vi "nanocal-frontend-server.vi"() -> ()   [LabVIEW 2020]
uses:
  icicle.ctl
  publisher action.ctl
  NanoCalLib 20210521/NanoCalLib.lvlibp
  NanoCalLib 20210521/MCL.lvlibp/SynkTek FPGA/FPGA_SharedResources/FPGASharedResources_Lockin_Typedef.ctl
  NanoCalLib 20210521/MCL.lvlibp/SynkTek FPGA/FPGA_SharedResources/FPGA_SharedResources.lvlib
  NanoCalLib 20210521/MCL.lvlibp
  NanoCalLib 20210521/MCL.lvlibp/SynkTek FPGA/FPGA_SharedResources/FPGASharedResources_Readings_ReadingChannelTypedef.ctl
  NanoCalLib 20210521/MCL.lvlibp/SynkTek FPGA/FPGA_SharedResources/FPGASharedResources_PhaseType_Typedef.ctl
panel:
  in  "Tab Control":enum32{"Page 1", "Page 2"}(tab)
  in  "wait (ms)":u32=50
  out "nanocal data":T1[](array[typedef])=[{"name"="frequency", "units"="Hz", "data"=22.999983439900642}, {"name"="Cs/T", "units"="J/K^2", "data"=3.7739249893269324e-24}, {"name"="Ts", "units"="K", "data"=0.01038672245174747}, {"name"="Ts^2", "units"="K^2", "data"=0.00010788400328963498}, {"name"="Tr", "units"="K", "data"=0.010160855980464388}, {"name"="Cs", "units"="J/K", "data"=3.9198711417852884e-26}, {"name"="Cr", "units"="J/K", "data"=-2.0417082109734875e-18}, {"name"="Ks", "units"="W/K", "data"=2.527872170547633e-23}, {"name"="Kr", "units"="W/K", "data"=3.911459306754245e-15}, {"name"="Rs-therm", "units"="Ohm", "data"=81348.62911437088}, {"name"="Rr-therm", "units"="Ohm", "data"=196009.13306498667}, {"name"="Cr/T", "units"="J/K^2", "data"=-2.0093860348960226e-16}, {"name"="dlogR/dlogT -- S ", "units"="a.u.", "data"=0.8738049990739949}, {"name"="tau", "units"="s", "data"=0.001550660348832471}, {"name"="tan(phi)", "units"="a.u", "data"=0.4481816480367121}, {"name"="Ts,ac", "units"="K", "data"=0.1660718459124116}, {"name"="Tr,ac", "units"="K", "data"=0.0}, {"name"="Hs,ac,out", "units"="V", "data"=0.0}, {"name"="Offset,dc,out", "units"="V", "data"=1.0000000009313226}, {"name"="Vdiff,ac", "units"="V", "data"=4.688238574611993e-09}, {"name"="Vdiff,ac,phase", "units"="deg", "data"=82.61397850464}, {"name"="Stherm,ac,out", "units"="V", "data"=0.0}, {"name"="Rtherm,ac,out", "units"="V", "data"=0.0}, {"name"="CV1 -- Re", "units"="V", "data"=6.026901987025408e-10}, {"name"="CV1 -- Im", "units"="V", "data"=4.649338174070346e-09}, {"name"="DV2 -- Re", "units"="V", "data"=1.0380460195223816e-09}, {"name"="DV2 -- Im", "units"="V", "data"=6.197949303499005e-09}, {"name"="AV2 -- Re", "units"="V", "data"=6.687727898351347e-10}, {"name"="AV2 -- Im", "units"="V", "data"=1.6238645509657183e-10}, {"name"="Vdiff,norm, Re", "units"="V", "data"=1.298136411917629e+18}, {"name"="Vdiff,norm, Im", "units"="V", "data"=1.00142248672243e+19}, {"name"="Resistance.RHr", "units"="ohm", "data"=501162.54690786166}, {"name"="Resistance.RHs", "units"="ohm", "data"=286805.4208747116}]
  in  "Stop":bool
  # "nanocal -- frontend server"
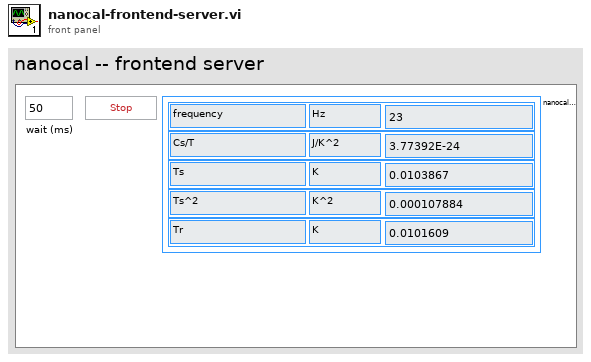
[diagram p1: front panel]
types:
  T1 = typedef "icicle.ctl" = cluster{"name":string, "units":string, "data":dbl}
  T2 = typedef "publisher action.ctl" = enum16{"set", "get", "init", "check"}
  T3 = typedef "MCL.lvlibp/FPGA_SharedResources.lvlib/FPGASharedResources_PhaseType_Typedef.ctl" = enum16{"DC", "X", "Y", "R", "Theta"}
  T4 = typedef "NanoCalLib.lvlibp/NanoReadings.lvlib/NanoReadings_Parameters_TypeDef.ctl" = cluster{"Power":T5, "C and K":T6, "IV dc":T7, "Tdc,Tac":T8, "Phases":T9, "f etc":T10, "IV 1st harm":T11, "ForAveraging":cluster{"SinTherm":dbl[], "CosTherm":dbl[], "SinHeats":dbl[], "CosHeats":dbl[]}, "Output":T12, "Magnetic field etc.":T13, "Calibration":T14, "CT etc":T15, "IV 2nd harm":T16, "Resistance":T17, "Time etc":T18}
  T5 = typedef "NanoCalLib.lvlibp/NanoReadings.lvlib/NanoReadings_Power.ctl" = cluster{"PHs (W)":dbl, "PHr (W)":dbl, "Ps,dc (W)":dbl, "Pr,dc (W)":dbl, "PHs,dc (W)":dbl, "PHr,dc (W)":dbl, "Ps,ac (W)":dbl, "Pr,ac (W)":dbl, "PHs/PHr":dbl, "Poffs (W)":dbl, "Ps total (W)":dbl, "Pr total (W)":dbl, "Ps-Pr total (W)":dbl, "Ps,offs (W)":dbl, "Ps,cond (W)":dbl, "Ps,net (W)":dbl}
  T6 = typedef "NanoCalLib.lvlibp/NanoReadings.lvlib/NanoReadings_CandK.ctl" = cluster{"Cs (J/K)":dbl, "Ks (W/K)":dbl, "Cr (J/K)":dbl, "Kr (W/K)":dbl, "Cdiff (J/K)":dbl, "Cs-Cr (J/K)":dbl, "Cdiff old style (J/K)":dbl, "Cr from S,diff (J/K)":dbl, "Cs from dT/dt (J/K)":dbl, "Ks,nom (W/K)":dbl}
  T7 = typedef "NanoCalLib.lvlibp/NanoReadings.lvlib/NanoReadings_IandV.ctl" = cluster{"Is,dc (A)":dbl, "Ir,dc (A)":dbl, "Us,dc (V)":dbl, "Ur,dc (V)":dbl, "Udiff,dc (V)":dbl, "IHs dc (A)":dbl, "UHs dc (V)":dbl, "IHr dc (A)":dbl, "UHr dc (V)":dbl, "Uoffs dc (V)":dbl, "Ioffs dc (A)":dbl}
  T8 = typedef "NanoCalLib.lvlibp/NanoReadings.lvlib/NanoReadings_TdcTac.ctl" = cluster{"Ts (K)":dbl, "Tr (K)":dbl, "Tdiff from Rs,Rr":dbl, "Tdiff from Udiff (K)":dbl, "Ts,ac (K)":dbl, "Tr,ac (K)":dbl, "Tdiff,ac (K)":dbl, "Ts,ac driftcorr (K)":dbl, "Tr,ac driftcorr (K)":dbl, "Tr,ac from Ts,diff,ac (K)":dbl, "T target (K)":dbl, "Ts^2 (K^2)":dbl, "Tr^2 (K^2)":dbl, "Tcos/(P/K)":dbl, "Tsin/(P/K)":dbl}
  T9 = typedef "NanoCalLib.lvlibp/NanoReadings.lvlib/NanoReadings_Phases.ctl" = cluster{"Phi Is (deg)":dbl, "Phi Us (deg)":dbl, "Phi Ir (deg)":dbl, "Phi Ur (deg)":dbl, "Phi Udiff (deg)":dbl, "Phi IHs (deg)":dbl, "Phi UHs (deg)":dbl, "Phi IHr (deg)":dbl, "Phi UHr (deg)":dbl, "Phi R from S,diff (deg)":dbl, "Phi Is 1st (deg)":dbl, "Phi Us 1st (deg)":dbl, "Phi Ir 1st (deg)":dbl, "Phi Ur 1st (deg)":dbl, "Phi Udiff 1st (deg)":dbl, "Phi Udiff, raw (deg)":dbl, "S phase (deg)":dbl, "R phase (deg)":dbl, "Diff phase (deg)":dbl}
  T10 = typedef "NanoCalLib.lvlibp/NanoReadings.lvlib/NanoReadings_Frequencies.ctl" = cluster{"f (Hz)":dbl, "f therm (Hz)":dbl, "omega (rad/s)":dbl, "Tan Phi S/diff":dbl, "Sin Phi":dbl, "Cos Phi":dbl, "f mix (Hz)":dbl, "tau (s)":dbl}
  T11 = typedef "NanoCalLib.lvlibp/NanoReadings.lvlib/NanoReadings_FirstHarmonic.ctl" = cluster{"Is,ac 1st (A)":dbl, "Ir,ac 1st (A)":dbl, "Us,ac 1st (V)":dbl, "Ur,ac 1st (V)":dbl, "Udiff,ac 1st (V)":dbl, "IHs (A)":dbl, "UHs (V)":dbl, "IHr (A)":dbl, "UHr (V)":dbl}
  T12 = typedef "NanoCalLib.lvlibp/NanoReadings.lvlib/NanoReadings_Output.ctl" = cluster{"S out phase (deg)":dbl, "R out phase (deg)":dbl, "Hs ac out (Vrms)":dbl, "Hr ac out (Vrms)":dbl, "S Therm dc out (V)":dbl, "R Therm dc out (V)":dbl, "S Therm ac out (Vrms)":dbl, "R Therm ac out (Vrms)":dbl, "Offset dc out (V)":dbl, "Hs dc out (V)":dbl, "Hr dc out (V)":dbl, "Offset ac out (Vrms)":dbl}
  T13 = typedef "NanoCalLib.lvlibp/NanoReadings.lvlib/NanoReadings_MagneticFieldEtc.ctl" = cluster{"H (T)":dbl, "T probe (K)":dbl, "Polar angle (deg)":dbl, "Azimuthal angle (deg)":dbl}
  T14 = typedef "NanoCalLib.lvlibp/NanoReadings.lvlib/NanoReadings_Calibration.ctl" = cluster{"1+Rs/RIs factor":dbl, "1+RIs/Rs factor":dbl, "Rs,scaled (ohm)":dbl, "Rr,scaled (ohm)":dbl, "R lead S (ohm)":dbl, "R lead R (ohm)":dbl, "|dlnR/dlnT| S":dbl, "|dlnR/dlnT| R":dbl, "dTs/dt (mK/s)":dbl, "dTr/dt (mK/s)":dbl}
  T15 = typedef "NanoCalLib.lvlibp/NanoReadings.lvlib/NanoReadings_CTetc.ctl" = cluster{"Cs/T (J/K^2)":dbl, "Cr/T (J/K^2)":dbl, "Cdiff/T (J/K^2)":dbl, "(Cs-Cr)/T (J/K^2)":dbl, "Cdiff/T old style (J/K^2)":dbl, "Cr/T from S,diff (J/K^2)":dbl}
  T16 = typedef "NanoCalLib.lvlibp/NanoReadings.lvlib/NanoReadings_2ndHarmonic.ctl" = cluster{"Is,ac (A)":dbl, "Ir,ac (A)":dbl, "Us,ac (V)":dbl, "Ur,ac (V)":dbl, "Udiff,ac (V)":dbl}
  T17 = typedef "NanoCalLib.lvlibp/NanoReadings.lvlib/NanoReadings_Resistance.ctl" = cluster{"RHs (ohm)":dbl, "RHr (ohm)":dbl, "Rs (ohm)":dbl, "Rr (ohm)":dbl, "RHs,dc (ohm)":dbl, "RHr,dc (ohm)":dbl, "Rs,ac (ohm)":dbl, "Rr,ac (ohm)":dbl, "Roffs (ohm)":dbl}
  T18 = typedef "NanoCalLib.lvlibp/NanoReadings.lvlib/NanoReadings_TimeEtc.ctl" = cluster{"Time (s)":dbl, "Datapoint index":dbl, "Datapoint time (s)":dbl}
  T19 = typedef "MCL.lvlibp/FPGA_SharedResources.lvlib/FPGASharedResources_Lockin_Typedef.ctl" = enum8{"Lock-in set L1", "Lock-in set L2"}
  T20 = typedef "MCL.lvlibp/FPGA_SharedResources.lvlib/FPGASharedResources_Readings_ReadingChannelTypedef.ctl" = enum8{"A V1", "A V2", "B V1", "B V2", "C V1", "C V2", "D V1", "D V2", "E V1", "E V2", "A I", "B I", "C I", "D I", "E I", "Int."}
  T21 = typedef "MCL.lvlibp/MCL_DataRef.ctl" = refnum<vi>
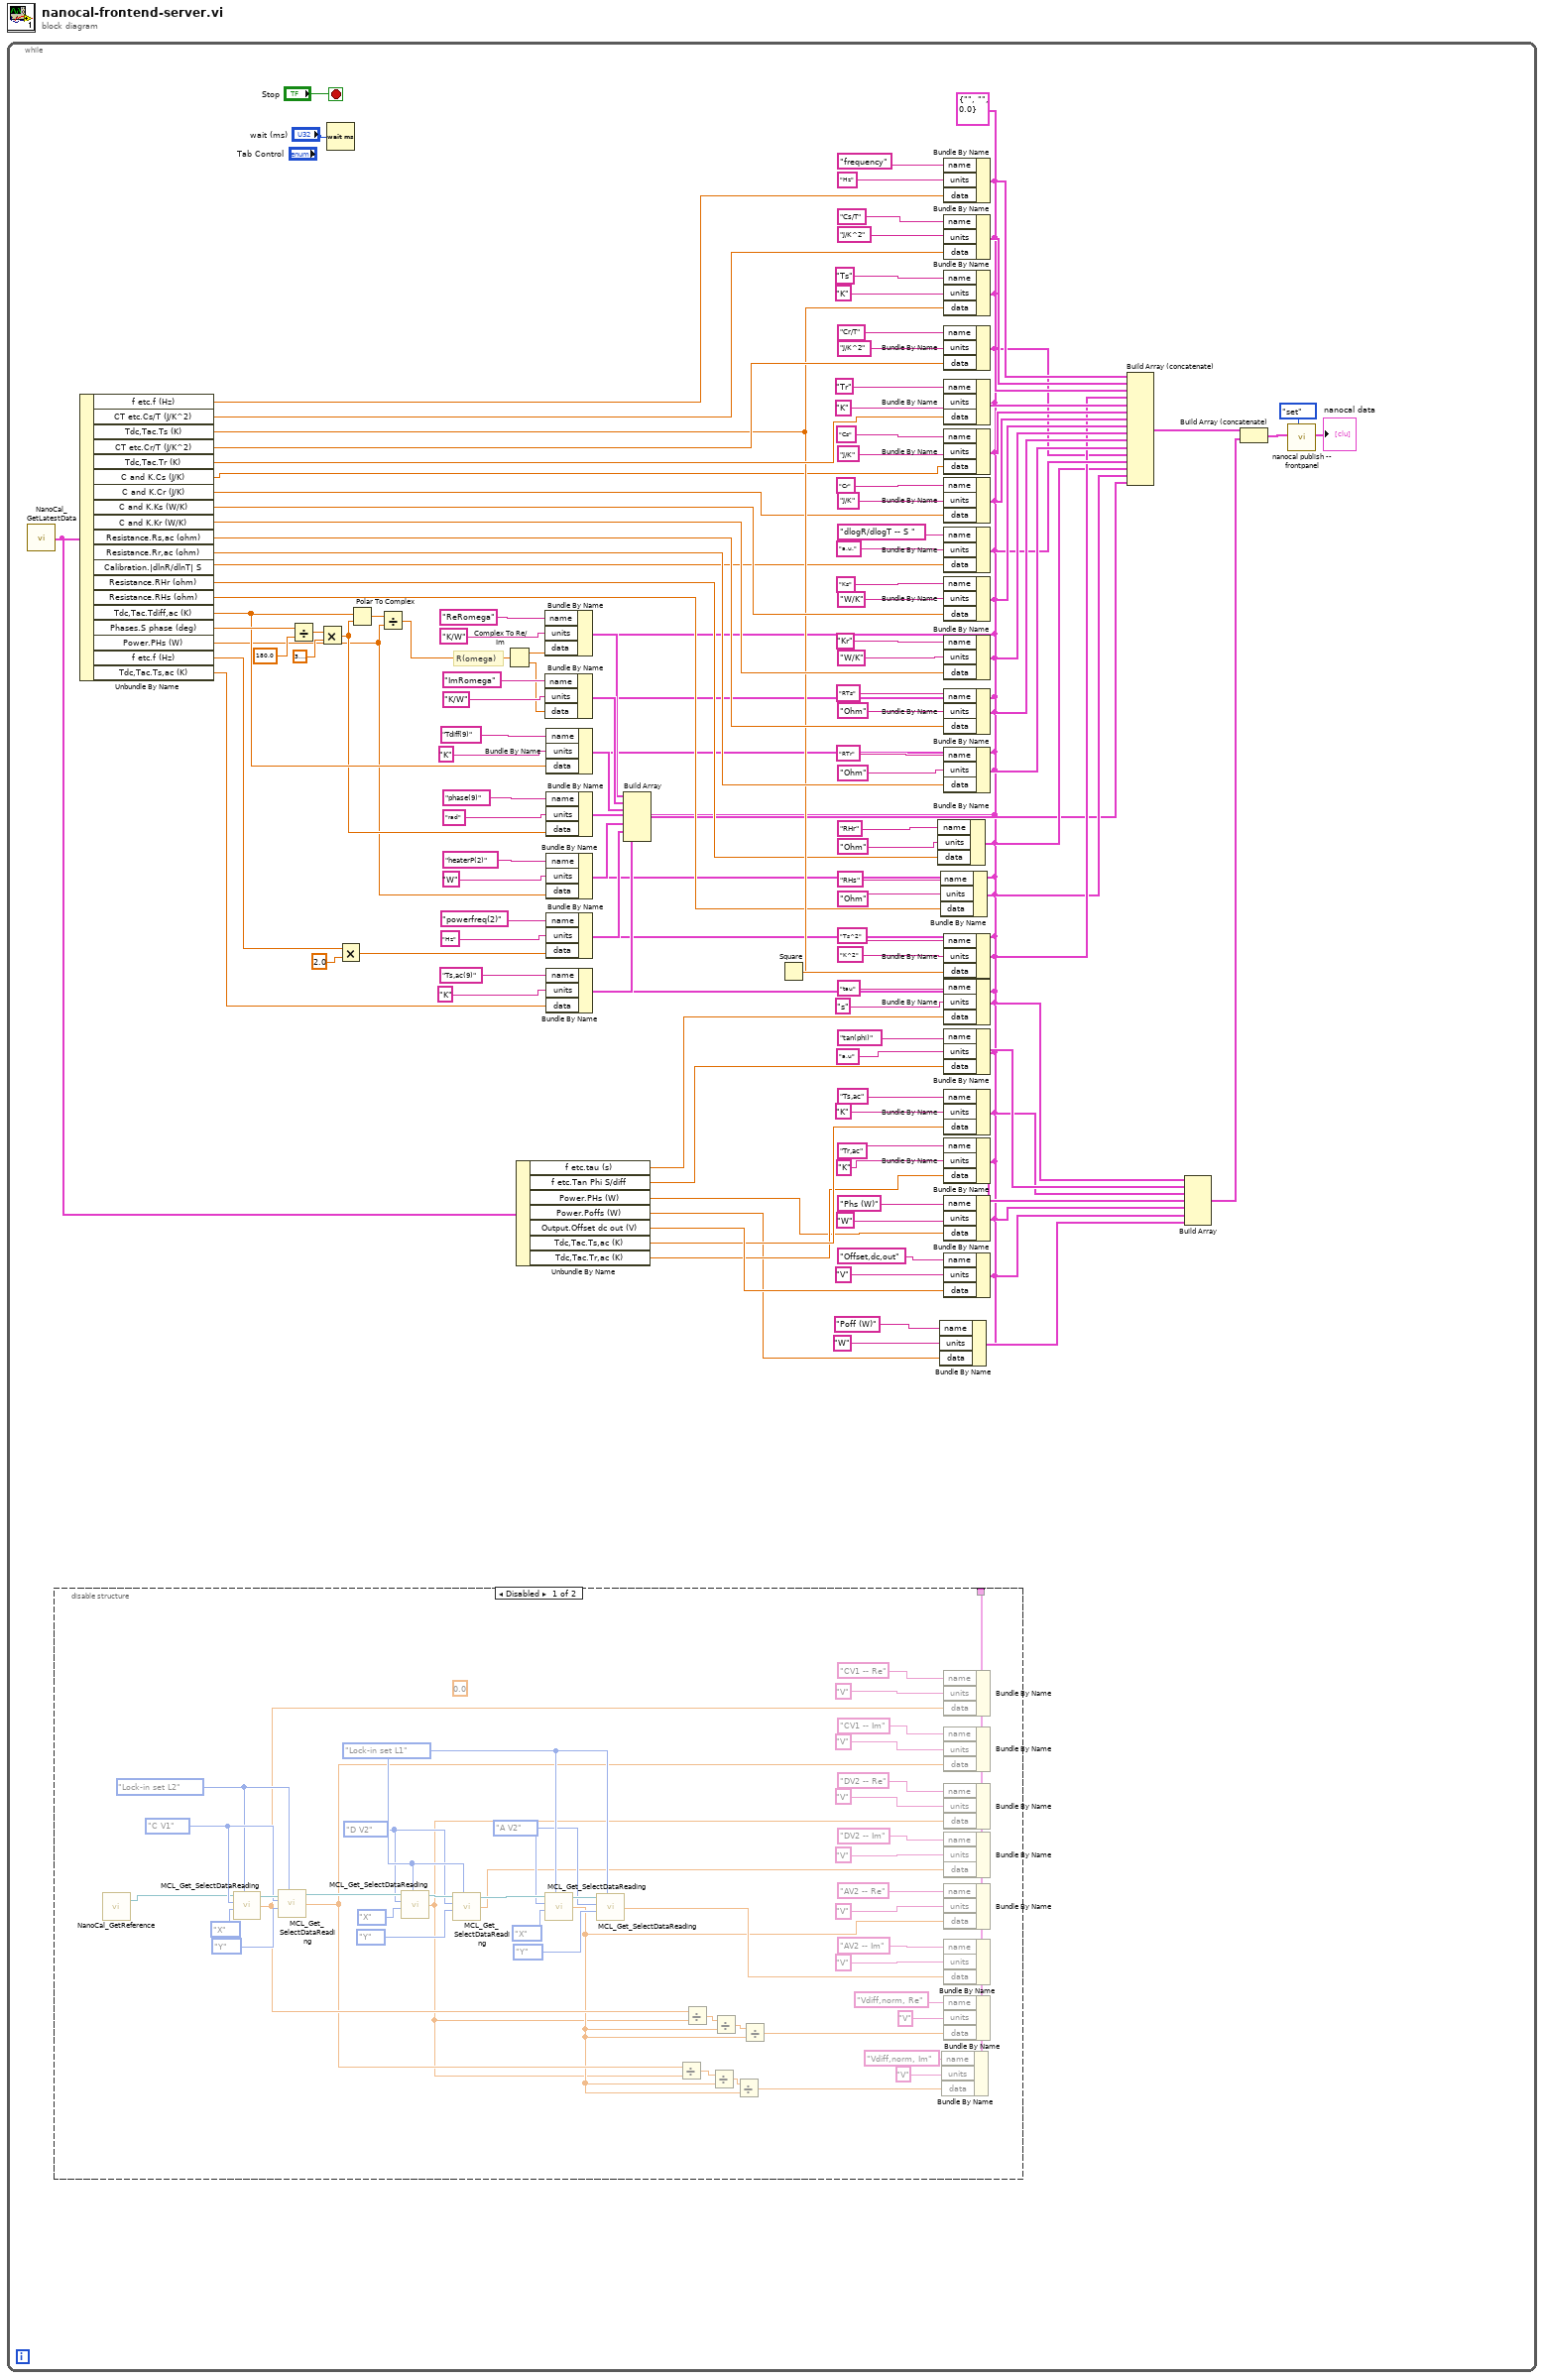
[diagram p0: block diagram]
diagram:
  n1 = while {
    stop <- "Stop" stop-if-true
    w1 = T1 {"name"="", "units"="", "data"=0.0} ("icicle")
    # "R(omega)"
    n2 = call "NanoCal_GetLatestData.vi"() -> ("Latest data"=w52:T4)  [unwired: 1 in]
    n3 = disable-structure shown="Disabled" {
      disable-tunnel: _ -> [w136 _]
      frame Disabled {
        w171 = FPGASharedResources_Lockin_Typedef."Lock-in set L1" ("Lockin")
        w168 = FPGASharedResources_Readings_ReadingChannelTypedef."A V2" ("Reading Ch")
        w167 = FPGASharedResources_Readings_ReadingChannelTypedef."D V2" ("Reading Ch")
        w178 = FPGASharedResources_Lockin_Typedef."Lock-in set L2" ("Lockin")
        w179 = FPGASharedResources_Readings_ReadingChannelTypedef."C V1" ("Reading Ch")
        (unwired) 0.0 ("Select reading")
        n4 = call "NanoCal_GetReference.vi"() -> ("Connected MCL object"=w135:T21)  [unwired: 2 in, 1 out]
        n5 = call "MCL_Get_SelectDataReading.vi"("MCL object"=w135, "Reading Ch"=w179, "PhaseType"=FPGASharedResources_PhaseType_Typedef."X", "Lockin"=w178) -> ("MCL object"=w180:T21, "Select reading"=w148:dbl)  [unwired: 1 in, 1 out]
        n6 = call "MCL_Get_SelectDataReading.vi"("MCL object"=w180, "Reading Ch"=w179, "PhaseType"=FPGASharedResources_PhaseType_Typedef."Y", "Lockin"=w178) -> ("MCL object"=w175:T21, "Select reading"=w142:dbl)  [unwired: 1 in, 1 out]
        n7 = call "MCL_Get_SelectDataReading.vi"("MCL object"=w175, "Reading Ch"=w167, "PhaseType"=FPGASharedResources_PhaseType_Typedef."X", "Lockin"=w171) -> ("MCL object"=w174:T21, "Select reading"=w139:dbl)  [unwired: 1 in, 1 out]
        n8 = call "MCL_Get_SelectDataReading.vi"("MCL object"=w174, "Reading Ch"=w167, "PhaseType"=FPGASharedResources_PhaseType_Typedef."Y", "Lockin"=w171) -> ("MCL object"=w173:T21, "Select reading"=w153:dbl)  [unwired: 1 in, 1 out]
        n9 = call "MCL_Get_SelectDataReading.vi"("MCL object"=w173, "Reading Ch"=w168, "PhaseType"=FPGASharedResources_PhaseType_Typedef."X", "Lockin"=w171) -> ("MCL object"=w172:T21, "Select reading"=w140:dbl)  [unwired: 1 in, 1 out]
        n10 = call "MCL_Get_SelectDataReading.vi"("MCL object"=w172, "Reading Ch"=w168, "PhaseType"=FPGASharedResources_PhaseType_Typedef."Y", "Lockin"=w171) -> ("Select reading"=w154:dbl)  [unwired: 1 in, 2 out]
        n11 = Divide(x=w142, y=w139) -> (x/y=w144:dbl)
        n12 = Divide(x=w148, y=w139) -> (x/y=w147:dbl)
        n13 = Divide(x=w144, y=w140) -> (x/y=w143:dbl)
        n14 = Divide(x=w147, y=w140) -> (x/y=w146:dbl)
        n15 = Divide(x=w143, y=w140) -> (x/y=w141:dbl)
        n16 = Divide(x=w146, y=w140) -> (x/y=w145:dbl)
        n17 = Bundle By Name(cluster=w136, "name"="Vdiff,norm, Im", "units"="V", "data"=w141) -> (w137:cluster{})
        n18 = Bundle By Name(cluster=w136, "name"="CV1 -- Re", "units"="V", "data"=w148) -> (w184:cluster{})
        n19 = Bundle By Name(cluster=w136, "name"="CV1 -- Im", "units"="V", "data"=w142) -> (w183:cluster{})
        n20 = Bundle By Name(cluster=w136, "name"="DV2 -- Re", "units"="V", "data"=w139) -> (w158:cluster{})
        n21 = Bundle By Name(cluster=w136, "name"="DV2 -- Im", "units"="V", "data"=w153) -> (w157:cluster{})
        n22 = Bundle By Name(cluster=w136, "name"="AV2 -- Re", "units"="V", "data"=w140) -> (w156:cluster{})
        n23 = Bundle By Name(cluster=w136, "name"="AV2 -- Im", "units"="V", "data"=w154) -> (w155:cluster{})
        n24 = Bundle By Name(cluster=w136, "name"="Vdiff,norm, Re", "units"="V", "data"=w145) -> (w138:cluster{})
      }
      frame Enabled {
      }
    }
    n25 = Unbundle By Name(w52) -> ("f etc.f (Hz)"=w129:dbl, "CT etc.Cs/T (J/K^2)"=w121:dbl, "Tdc,Tac.Ts (K)"=w93:dbl, "CT etc.Cr/T (J/K^2)"=w122:dbl, "Tdc,Tac.Tr (K)"=w116:dbl, "C and K.Cs (J/K)"=w87:dbl, "C and K.Cr (J/K)"=w86:dbl, "C and K.Ks (W/K)"=w112:dbl, "C and K.Kr (W/K)"=w106:dbl, "Resistance.Rs,ac (ohm)"=w98:dbl, "Resistance.Rr,ac (ohm)"=w97:dbl, "Calibration.|dlnR/dlnT| S"=w56:dbl, "Resistance.RHr (ohm)"=w47:dbl, "Resistance.RHs (ohm)"=w46:dbl, "Tdc,Tac.Tdiff,ac (K)"=w27:dbl, "Phases.S phase (deg)"=w42:dbl, "Power.PHs (W)"=w23:dbl, "f etc.f (Hz)"=w20:dbl, "Tdc,Tac.Ts,ac (K)"=w2:dbl)
    n26 = Divide(x=w42, y=180.0) -> (x/y=w43:dbl)
    n27 = Multiply(x=w43, y=3.141592653589793) -> (x*y=w26:dbl)
    n28 = Wait (ms)(milliseconds to wait="wait (ms)") -> ()  [unwired: 1 out]
    n29 = Multiply(x=w20, y=2.0) -> (x*y=w18:dbl)
    n30 = Polar To Complex(1:w26, 2:w27) -> (0:w39:cdb)
    n31 = Divide(x=w39, y=w23) -> (x/y=w34:cdb)
    n32 = Complex To Re/Im(x + iy=w34) -> (x=w33:dbl, y=w32:dbl)
    n33 = Unbundle By Name(w52) -> ("f etc.tau (s)"=w76:dbl, "f etc.Tan Phi S/diff"=w68:dbl, "Power.PHs (W)"=w10:dbl, "Power.Poffs (W)"=w6:dbl, "Output.Offset dc out (V)"=w73:dbl, "Tdc,Tac.Ts,ac (K)"=w72:dbl, "Tdc,Tac.Tr,ac (K)"=w71:dbl)
    n34 = Bundle By Name(cluster=w1, "name"="ReRomega", "units"="K/W", "data"=w33) -> (w16:T1)
    n35 = Bundle By Name(cluster=w1, "name"="ImRomega", "units"="K/W", "data"=w32) -> (w17:T1)
    n36 = Bundle By Name(cluster=w1, "name"="Tdiff(9)", "units"="K", "data"=w27) -> (w15:T1)
    n37 = Bundle By Name(cluster=w1, "name"="phase(9)", "units"="rad", "data"=w26) -> (w14:T1)
    n38 = Bundle By Name(cluster=w1, "name"="heaterP(2)", "units"="W", "data"=w23) -> (w13:T1)
    n39 = Bundle By Name(cluster=w1, "name"="powerfreq(2)", "units"="Hz", "data"=w18) -> (w12:T1)
    n40 = Bundle By Name(cluster=w1, "name"="Ts,ac(9)", "units"="K", "data"=w2) -> (w3:T1)
    n41 = Build Array(w16, w17, w15, w14, w13, w12, w3) -> (w11:T1[])
    n42 = Square(x=w93) -> (x^2=w94:dbl)
    n43 = Bundle By Name(cluster=w1, "name"="RHr", "units"="Ohm", "data"=w47) -> (w45:T1)
    n44 = Bundle By Name(cluster=w1, "name"="Poff (W)", "units"="W", "data"=w6) -> (w7:T1)
    n45 = Bundle By Name(cluster=w1, "name"="RHs", "units"="Ohm", "data"=w46) -> (w44:T1)
    n46 = Bundle By Name(cluster=w1, "name"="frequency", "units"="Hz", "data"=w129) -> (w118:T1)
    n47 = Bundle By Name(cluster=w1, "name"="Cs/T", "units"="J/K^2", "data"=w121) -> (w119:T1)
    n48 = Bundle By Name(cluster=w1, "name"="Ts", "units"="K", "data"=w93) -> (w120:T1)
    n49 = Bundle By Name(cluster=w1, "name"="Cr/T", "units"="J/K^2", "data"=w122) -> (w53:T1)
    n50 = Bundle By Name(cluster=w1, "name"="Tr", "units"="K", "data"=w116) -> (w115:T1)
    n51 = Bundle By Name(cluster=w1, "name"="Cs", "units"="J/K", "data"=w87) -> (w90:T1)
    n52 = Bundle By Name(cluster=w1, "name"="Cr", "units"="J/K", "data"=w86) -> (w85:T1)
    n53 = Bundle By Name(cluster=w1, "name"="dlogR/dlogT -- S ", "units"="a.u.", "data"=w56) -> (w55:T1)
    n54 = Bundle By Name(cluster=w1, "name"="Ks", "units"="W/K", "data"=w112) -> (w111:T1)
    n55 = Bundle By Name(cluster=w1, "name"="Kr", "units"="W/K", "data"=w106) -> (w105:T1)
    n56 = Bundle By Name(cluster=w1, "name"="RTs", "units"="Ohm", "data"=w98) -> (w100:T1)
    n57 = Bundle By Name(cluster=w1, "name"="RTr", "units"="Ohm", "data"=w97) -> (w99:T1)
    n58 = Bundle By Name(cluster=w1, "name"="Ts^2", "units"="K^2", "data"=w94) -> (w54:T1)
    n59 = Bundle By Name(cluster=w1, "name"="tau", "units"="s", "data"=w76) -> (w67:T1)
    n60 = Bundle By Name(cluster=w1, "name"="tan(phi)", "units"="a.u", "data"=w68) -> (w66:T1)
    n61 = Bundle By Name(cluster=w1, "name"="Ts,ac", "units"="K", "data"=w72) -> (w65:T1)
    n62 = Bundle By Name(cluster=w1, "name"="Tr,ac", "units"="K", "data"=w71) -> (w64:T1)
    n63 = Bundle By Name(cluster=w1, "name"="Phs (W)", "units"="W", "data"=w10) -> (w63:T1)
    n64 = Bundle By Name(cluster=w1, "name"="Offset,dc,out", "units"="V", "data"=w73) -> (w62:T1)
    n65 = Build Array (concatenate)(w118, w119, w120, w54, w115, w90, w85, w111, w105, w100, w99, w53, w55, w45, w44, w11) -> (w61:T1[])
    n66 = Build Array(w67, w66, w65, w64, w63, w62, w7) -> (w60:T1[])
    n67 = Build Array (concatenate)(w61, w60) -> (w59:T1[])
    n68 = call "nanocal publish -- frontpanel.vi"("publisher action"=publisher_action."set", "nanocal data array IN"=w59) -> ("nanocal data array OUT"=→"nanocal data":T1[])  [unwired: 9 in]
  }
